vi "Write SnP File.vi"(5 "OutputDataType":T1=enum."RI", 6 "Z0 (50 Ohm)":dbl=50.0, 7 "Comments":string[](array[string]), 8 "error in (no error)":errorcluster, 9 "S-parameters":cdb[][](array[numeric]), 10 "Frequencies (Hz)":dbl[](array[numeric]), 11 "SnP File Path":path) -> (0 "error out":errorcluster)   [LabVIEW 2023, in "NI_HFNetworkAnalysis.lvlib"]
doc: "Writes S-parameters to the specified file using the Touchstone File Format specifications.\n\n<b>Requirements</B>\nThe directory specified as part of the file name is assumed to exist.\n\n<b>Note</b>\nIf the reference SnP file already exists, it will be overwritten."
uses:
  NI_HFNetworkAnalysis.lvlib
  Controls/SnPDataType.ctl
  C:/srd-semi-rfcal-software/AuxTools/STSRFFixtureCharactUtility/Source/Code Modules/Fixture/Dependencies/HFNetworkAnalysis/Support Files/NACE.Utils.Data.dll
  Support Files/NACE.Utils.Data.dll
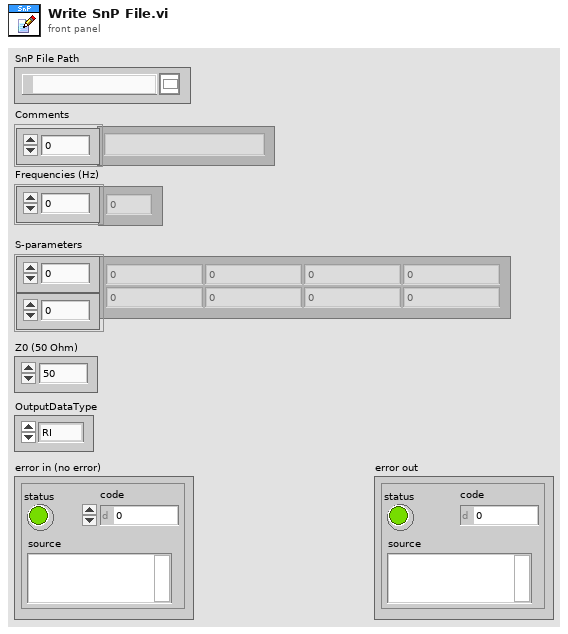
[diagram p1: front panel]
types:
  T1 = typedef "NI_HFNetworkAnalysis.lvlib/SnPDataType.ctl" = enum16{"DB", "MA", "RI"}
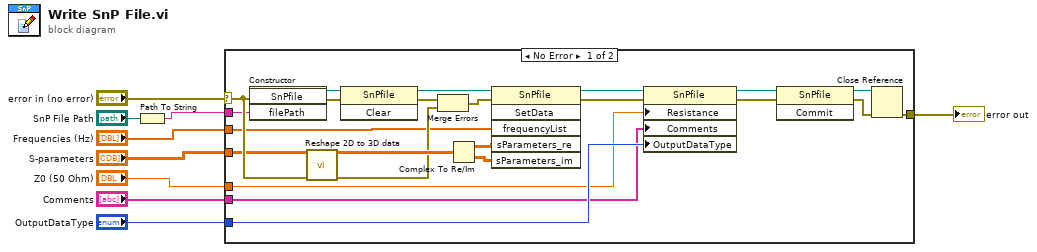
[diagram p0: block diagram]
diagram:
  n1 = Path To String(path="SnP File Path") -> (string=w2:string)
  n2 = case shown="No Error" "error in (no error)" {
    selector: "error in (no error)" -> [w22 w33]
    tunnel: [w29 w33] -> w9
    tunnel: w2 -> [w10 _]
    tunnel: "Frequencies (Hz)" -> [w20 _]
    tunnel: "S-parameters" -> [w21 _]
    tunnel: "Z0 (50 Ohm)" -> [w13 _]
    tunnel: "Comments" -> [w14 _]
    tunnel: "OutputDataType" -> [w19 _]
    frame No Error {
      n3 = constructor class="SnPfile"(error in=w22, "filePath"=w10) -> (reference out=w12:refnum<k24>, error out=w11:errorcluster)  [unwired: 2 in, 2 out]
      n4 = call "Reshape 2D to 3D data.vi"("Parameters In (2D)"=w21, "Error In"=w22) -> ("Parameters Out (3D)"=w26:cdb[][][], "Error Out"=w23:errorcluster)  [unwired: 12 in]
      n5 = invoke class="SnPfile" method="Clear"(reference=w12, error in=w11) -> (reference out=w30:refnum<k24>, error out=w25:errorcluster)  [unwired: 1 in, 1 out]
      n6 = Merge Errors(w25, w23) -> (w24:errorcluster)
      n7 = Complex To Re/Im(x + iy=w26) -> (x=w28:dbl[][][], y=w27:dbl[][][])
      n8 = invoke class="SnPfile" method="SetData"(reference=w30, error in=w24, "frequencyList"=w20, "sParameters_re"=w28, "sParameters_im"=w27) -> (reference out=w16:refnum<k24>, error out=w15:errorcluster)  [unwired: 1 in, 4 out]
      n9 = property class="SnPfile"(reference=w16, error in=w15, "Resistance"=w13, "Comments"=w14, "OutputDataType"=w19) -> (reference out=w18:refnum<k24>, error out=w17:errorcluster)
      n10 = invoke class="SnPfile" method="Commit"(reference=w18, error in=w17) -> (reference out=w32:refnum<k24>, error out=w31:errorcluster)  [unwired: 1 in, 1 out]
      n11 = Close Reference(reference=w32, error in (no error)=w31) -> (error out=w29:errorcluster)
    }
    frame Error {
    }
  }
  "error out" <- w9
